vi "核查数据时间戳转换 (子VI).vi"(10 "枚举":enum16{"零点跨度", "标样核查"}(ring), 11 "核查索引":string[](array[string])) -> (3 "数组":string[](array[string]))   [LabVIEW 2016, in "数据传输系统-05.lvlib"]
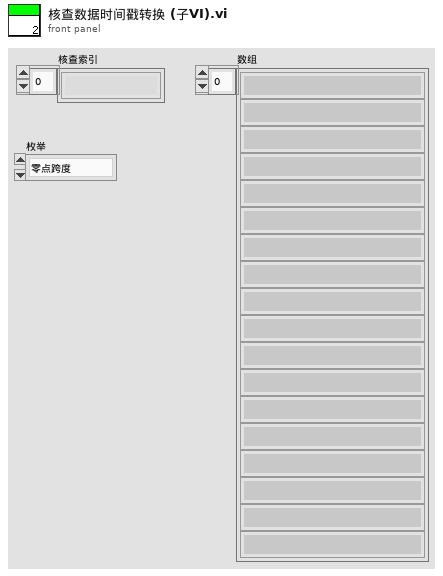
[diagram p1: front panel]
types:
  T1 = typedef "LVDateTimeRec.ctl" = cluster{"秒数的小数部分":dbl, "秒":i32, "分":i32, "时":i32, "日":i32, "月":i32, "年":i32, "天数（周）":i32, "天数（年）":i32, "DST":i32}
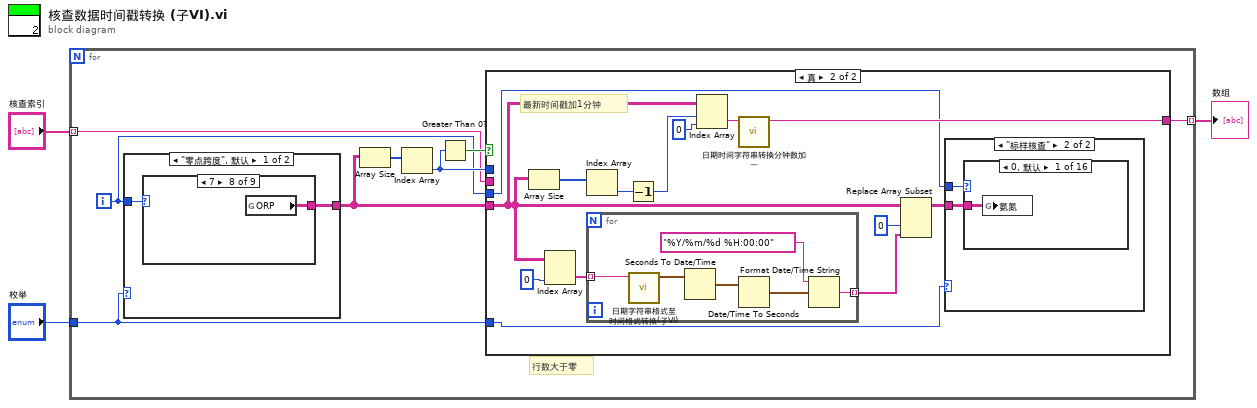
[diagram p0: block diagram]
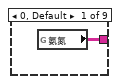
[diagram p2: hidden frame]
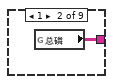
[diagram p3: hidden frame]
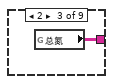
[diagram p4: hidden frame]
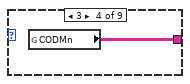
[diagram p5: hidden frame]
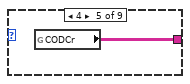
[diagram p6: hidden frame]
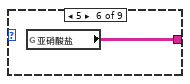
[diagram p7: hidden frame]
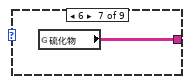
[diagram p8: hidden frame]
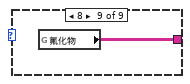
[diagram p9: hidden frame]
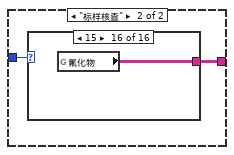
[diagram p10: hidden frame]
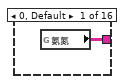
[diagram p11: hidden frame]
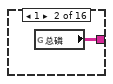
[diagram p12: hidden frame]
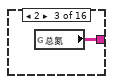
[diagram p13: hidden frame]
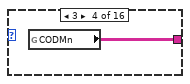
[diagram p14: hidden frame]
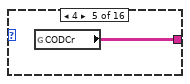
[diagram p15: hidden frame]
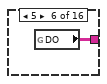
[diagram p16: hidden frame]
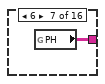
[diagram p17: hidden frame]
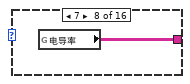
[diagram p18: hidden frame]
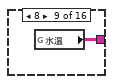
[diagram p19: hidden frame]
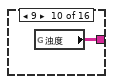
[diagram p20: hidden frame]
diagram:
  n1 = for {
    tunnel: [w8] -> w3 mode=indexing
    tunnel: "核查索引" -> [w7] mode=indexing
    tunnel: "枚举" -> [w4]
    i -> [w6]
    # "行数大于零"
    n2 = case shown="\"零点跨度\", 默认" w4 {
      tunnel: w6 -> [w12 w24]
      tunnel: [w13 w23] -> w5
      frame "零点跨度", Default {
        n3 = case shown="7" w12 {
          tunnel: [w14 w15 w16 w17 w18 w19 w20 w21 w22] -> w13
          frame 0, Default {
            n4 = global read "全局 所有参数.vi" "氨氮"() -> (w14:string[][])
          }
          frame 1 {
            n5 = global read "全局 所有参数.vi" "总磷"() -> (w15:string[][])
          }
          frame 2 {
            n6 = global read "全局 所有参数.vi" "总氮"() -> (w16:string[][])
          }
          frame 3 {
            n7 = global read "全局 所有参数.vi" "CODMn"() -> (w17:string[][])
          }
          frame 4 {
            n8 = global read "全局 所有参数.vi" "CODCr"() -> (w18:string[][])
          }
          frame 5 {
            n9 = global read "全局 所有参数.vi" "亚硝酸盐"() -> (w19:string[][])
          }
          frame 6 {
            n10 = global read "全局 所有参数.vi" "硫化物"() -> (w20:string[][])
          }
          frame 7 {
            n11 = global read "全局 所有参数.vi" "ORP"() -> (w21:string[][])
          }
          frame 8 {
            n12 = global read "全局 所有参数.vi" "氟化物"() -> (w22:string[][])
          }
        }
      }
      frame "标样核查" {
        n13 = case shown="15" w24 {
          tunnel: [w25 w26 w27 w28 w29 w30 w31 w32 w33 w34 w35 w36 w37 w38 w39 w40] -> w23
          frame 0, Default {
            n14 = global read "全局 所有参数.vi" "氨氮"() -> (w25:string[][])
          }
          frame 1 {
            n15 = global read "全局 所有参数.vi" "总磷"() -> (w26:string[][])
          }
          frame 2 {
            n16 = global read "全局 所有参数.vi" "总氮"() -> (w27:string[][])
          }
          frame 3 {
            n17 = global read "全局 所有参数.vi" "CODMn"() -> (w28:string[][])
          }
          frame 4 {
            n18 = global read "全局 所有参数.vi" "CODCr"() -> (w29:string[][])
          }
          frame 5 {
            n19 = global read "全局 所有参数.vi" "DO"() -> (w30:string[][])
          }
          frame 6 {
            n20 = global read "全局 所有参数.vi" "PH"() -> (w31:string[][])
          }
          frame 7 {
            n21 = global read "全局 所有参数.vi" "电导率"() -> (w32:string[][])
          }
          frame 8 {
            n22 = global read "全局 所有参数.vi" "水温"() -> (w33:string[][])
          }
          frame 9 {
            n23 = global read "全局 所有参数.vi" "浊度"() -> (w34:string[][])
          }
          frame 10 {
            n24 = global read "全局 所有参数.vi" "叶绿素"() -> (w35:string[][])
          }
          frame 11 {
            n25 = global read "全局 所有参数.vi" "藻密度"() -> (w36:string[][])
          }
          frame 12 {
            n26 = global read "全局 所有参数.vi" "亚硝酸盐"() -> (w37:string[][])
          }
          frame 13 {
            n27 = global read "全局 所有参数.vi" "硫化物"() -> (w38:string[][])
          }
          frame 14 {
            n28 = global read "全局 所有参数.vi" "ORP"() -> (w39:string[][])
          }
          frame 15 {
            n29 = global read "全局 所有参数.vi" "氟化物"() -> (w40:string[][])
          }
        }
      }
    }
    n30 = Array Size(array=w5) -> (size(s)=w10:i32[])
    n31 = Index Array(array=w10) -> (element=w9:i32)  [unwired: 1 in]
    n32 = Greater Than 0?(x=w9) -> (x > 0?=w11:bool)
    n33 = case shown="真" w11 {
      tunnel: w9 -> [_ _]
      tunnel: w5 -> [_ w47]
      tunnel: [w41 w51] -> w8
      tunnel: w7 -> [w41 _]
      tunnel: w6 -> [_ w43]
      tunnel: w4 -> [_ w42]
      frame False {
      }
      frame True {
        # "最新时间戳加1分钟"
        n34 = Array Size(array=w47) -> (size(s)=w55:i32[])
        n35 = Index Array(array=w47, index (col)=0 ("禁用的索引 (列)")) -> (element=w48:string[])  [unwired: 1 in]
        n36 = Index Array(array=w55) -> (element=w54:i32)  [unwired: 1 in]
        n37 = for {
          tunnel: w48 -> [w86] mode=indexing
          tunnel: [w85] -> w45 mode=indexing
          n38 = call "日期字符串格式至时间格式转换(子VI).vi"("data[0]"=w86) -> ("time stamp"=w88:timestamp)  [unwired: 10 in]
          n39 = Seconds To Date/Time(time stamp (now)=w88) -> (date time rec=w87:T1)  [unwired: 1 in]
          n40 = Date/Time To Seconds(2:w87) -> (0:w89:timestamp)  [unwired: 1 in]
          n41 = Format Date/Time String(time format string (%c)="%Y/%m/%d %H:00:00" ("时间格式字符串(%c)"), seconds (now)=w89) -> (date/time string=w85:string)  [unwired: 1 in]
        }
        n42 = Decrement(x=w54) -> (x-1=w53:i32)
        n43 = Index Array(array=w47, index (row)=w53, index (col)=0 ("禁用的索引 (列)")) -> (element=w50:string)
        n44 = call "日期时间字符串转换分钟数加一.vi"("data[0]"=w50) -> ("日期/时间字符串"=w51:string)  [unwired: 10 in]
        n45 = Replace Array Subset(array=w47, new element=w45, index (col)=0 ("禁用的索引 (列)")) -> (w44:string[][])  [unwired: 1 in]
        n46 = case shown="\"标样核查\"" w42 {
          tunnel: w43 -> [w56 w68]
          tunnel: w44 -> [w57 w67]
          frame "零点跨度", Default {
            n47 = case shown="8" w56 {
              tunnel: w57 -> [w58 w59 w60 w61 w62 w63 w64 w65 w66]
              frame 0, Default {
                n48 = global write "全局 所有参数.vi" "氨氮"(w58) -> ()
              }
              frame 1 {
                n49 = global write "全局 所有参数.vi" "总磷"(w59) -> ()
              }
              frame 2 {
                n50 = global write "全局 所有参数.vi" "总氮"(w60) -> ()
              }
              frame 3 {
                n51 = global write "全局 所有参数.vi" "CODMn"(w61) -> ()
              }
              frame 4 {
                n52 = global write "全局 所有参数.vi" "CODCr"(w62) -> ()
              }
              frame 5 {
                n53 = global write "全局 所有参数.vi" "亚硝酸盐"(w63) -> ()
              }
              frame 6 {
                n54 = global write "全局 所有参数.vi" "硫化物"(w64) -> ()
              }
              frame 7 {
                n55 = global write "全局 所有参数.vi" "ORP"(w65) -> ()
              }
              frame 8 {
                n56 = global write "全局 所有参数.vi" "氟化物"(w66) -> ()
              }
            }
          }
          frame "标样核查" {
            n57 = case shown="0, 默认" w68 {
              tunnel: w67 -> [w69 w70 w71 w72 w73 w74 w75 w76 w77 w78 w79 w80 w81 w82 w83 w84]
              frame 0, Default {
                n58 = global write "全局 所有参数.vi" "氨氮"(w69) -> ()
              }
              frame 1 {
                n59 = global write "全局 所有参数.vi" "总磷"(w70) -> ()
              }
              frame 2 {
                n60 = global write "全局 所有参数.vi" "总氮"(w71) -> ()
              }
              frame 3 {
                n61 = global write "全局 所有参数.vi" "CODMn"(w72) -> ()
              }
              frame 4 {
                n62 = global write "全局 所有参数.vi" "CODCr"(w73) -> ()
              }
              frame 5 {
                n63 = global write "全局 所有参数.vi" "DO"(w74) -> ()
              }
              frame 6 {
                n64 = global write "全局 所有参数.vi" "PH"(w75) -> ()
              }
              frame 7 {
                n65 = global write "全局 所有参数.vi" "电导率"(w76) -> ()
              }
              frame 8 {
                n66 = global write "全局 所有参数.vi" "水温"(w77) -> ()
              }
              frame 9 {
                n67 = global write "全局 所有参数.vi" "浊度"(w78) -> ()
              }
              frame 10 {
                n68 = global write "全局 所有参数.vi" "叶绿素"(w79) -> ()
              }
              frame 11 {
                n69 = global write "全局 所有参数.vi" "藻密度"(w80) -> ()
              }
              frame 12 {
                n70 = global write "全局 所有参数.vi" "亚硝酸盐"(w81) -> ()
              }
              frame 13 {
                n71 = global write "全局 所有参数.vi" "硫化物"(w82) -> ()
              }
              frame 14 {
                n72 = global write "全局 所有参数.vi" "ORP"(w83) -> ()
              }
              frame 15 {
                n73 = global write "全局 所有参数.vi" "氟化物"(w84) -> ()
              }
            }
          }
        }
      }
    }
  }
  "数组" <- w3
